vi "Format_Request.vi"(8 "error in (no error)":errorcluster, 10 "Request":T1=enum."PATCH_MULTIPART", 11 "Request in":refnum<class "Request.lvclass">) -> (0 "error out":errorcluster, 3 "Request out":refnum<class "Request.lvclass">)   [LabVIEW 2016, in "Request.lvclass"]
uses:
  Request.lvclass
  PowerShell_Format/Request_Control.ctl
  Request.lvclass/Request.ctl
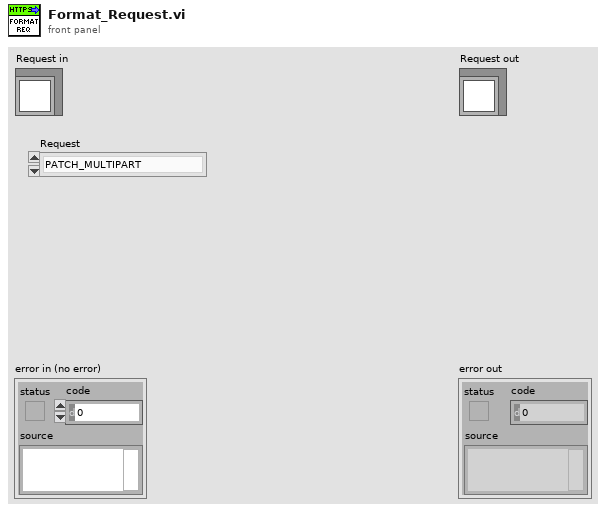
[diagram p1: front panel]
types:
  T1 = typedef "Request.lvclass/Request_Control.ctl" = enum16{"POST", "PATCH_MULTIPART", "POST_MULTIPART", "PATCH", "DELETE", "HEAD", "PUT", "GET"}
  T2 = cluster{"Name":string, "Value":string, "File":path, "Filename":string, "MIME type":string}[]
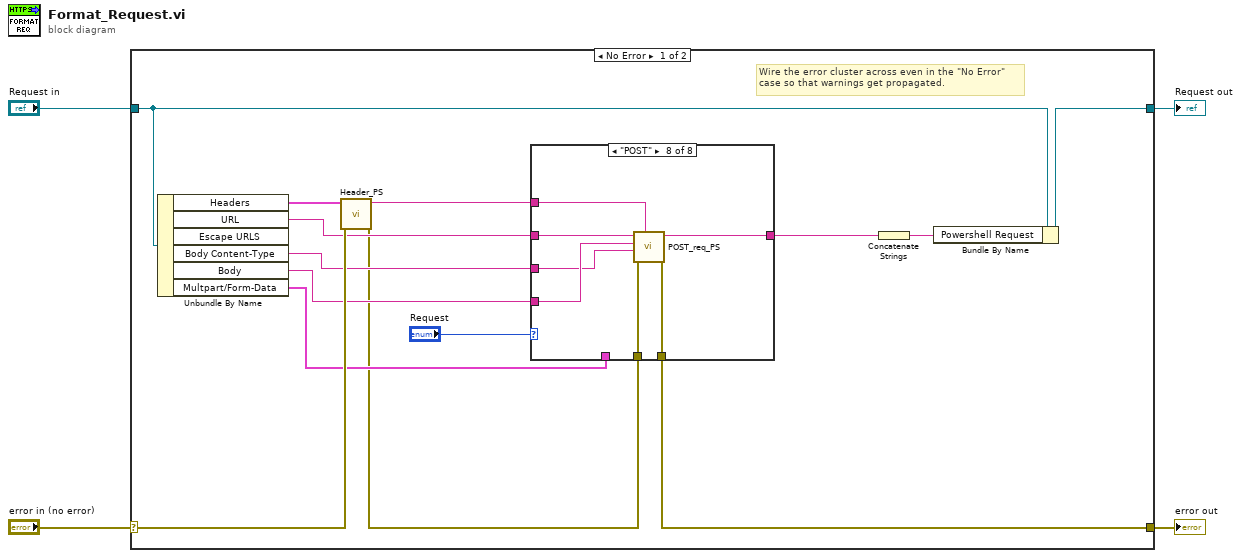
[diagram p0: block diagram]
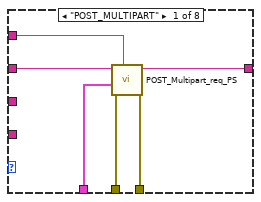
[diagram p2: hidden frame]
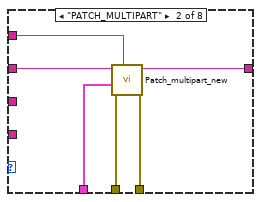
[diagram p3: hidden frame]
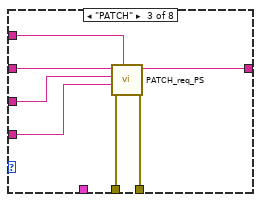
[diagram p4: hidden frame]
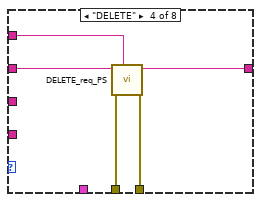
[diagram p5: hidden frame]
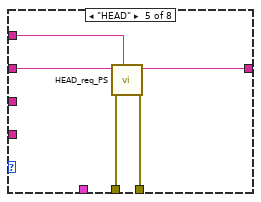
[diagram p6: hidden frame]
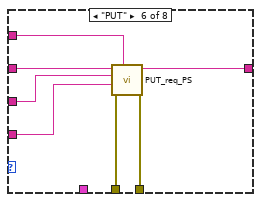
[diagram p7: hidden frame]
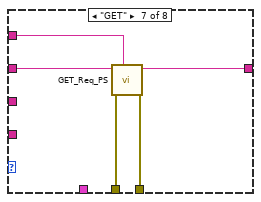
[diagram p8: hidden frame]
diagram:
  n1 = case shown="No Error" "error in (no error)" {
    selector: "error in (no error)" -> [w15 w68]
    tunnel: [w13 w68] -> w3
    tunnel: [w11 w67] -> w1
    tunnel: "Request in" -> [w12 w67]
    frame No Error {
      # "Wire the error cluster across even in the \"No Error\"\ncase so that warnings get propagated."
      n2 = Unbundle By Name(w12) -> ("Headers"=w14:cluster{"Name":string, "Value":string}[], "URL"=w9:string, "Body Content-Type"=w6:string, "Body"=w7:string, "Multpart/Form-Data"=w8:T2)  [unwired: 1 out]
      n3 = call "Header_PS.vi"("error in"=w15, "Headers In"=w14) -> ("error out"=w5:errorcluster, "Headers_PS_Dict"=w16:string)  [unwired: 8 in]
      n4 = case shown="\"POST\"" "Request" {
        tunnel: w8 -> [w24 w25 _ _ _ _ _ _]
        tunnel: w9 -> [w21 w29 w37 w39 w45 w54 w56 w62]
        tunnel: w5 -> [w23 w27 w36 w42 w47 w51 w57 w65]
        tunnel: [w22 w26 w35 w41 w46 w50 w58 w64] -> w13
        tunnel: w16 -> [w20 w30 w34 w38 w44 w49 w55 w63]
        tunnel: [w19 w28 w31 w40 w43 w48 w59 w66] -> w17
        tunnel: w6 -> [_ _ w32 _ _ w53 _ w60]
        tunnel: w7 -> [_ _ w33 _ _ w52 _ w61]
        frame "POST_MULTIPART" {
          n5 = call "POST_Multipart_req_PS.vi"("Headers"=w20, "error in"=w23, "Multpart/Form-Data"=w24, "URL"=w21) -> ("error out"=w22:errorcluster, "Multipart PATCH Request"=w19:string)  [unwired: 6 in]
        }
        frame "PATCH_MULTIPART" {
          n6 = call "Patch_multipart_new.vi"("Headers"=w30, "error in"=w27, "Multpart/Form-Data"=w25, "URL"=w29) -> ("error out"=w26:errorcluster, "Multipart PATCH Request"=w28:string)  [unwired: 6 in]
        }
        frame "PATCH" {
          n7 = call "PATCH_req_PS.vi"("Headers"=w34, "error in"=w36, "Body"=w33, "ContentType"=w32, "URL"=w37) -> ("error out"=w35:errorcluster, "PATCH Request"=w31:string)  [unwired: 5 in]
        }
        frame "DELETE" {
          n8 = call "DELETE_req_PS.vi"("Headers"=w38, "error in"=w42, "URL"=w39) -> ("error out"=w41:errorcluster, "DELETE Request"=w40:string)  [unwired: 7 in]
        }
        frame "HEAD" {
          n9 = call "HEAD_req_PS.vi"("Headers"=w44, "error in"=w47, "URL"=w45) -> ("error out"=w46:errorcluster, "HEAD Request"=w43:string)  [unwired: 7 in]
        }
        frame "PUT" {
          n10 = call "PUT_req_PS.vi"("Headers"=w49, "error in"=w51, "ContentType"=w52, "Body"=w53, "URL"=w54) -> ("error out"=w50:errorcluster, "PUT Request"=w48:string)  [unwired: 5 in]
        }
        frame "GET" {
          n11 = call "GET_Req_PS.vi"("Headers"=w55, "error in"=w57, "URL"=w56) -> ("error out"=w58:errorcluster, "GET Request"=w59:string)  [unwired: 7 in]
        }
        frame "POST" {
          n12 = call "POST_req_PS.vi"("Headers"=w63, "error in"=w65, "ContentType"=w60, "Body"=w61, "URL"=w62) -> ("error out"=w64:errorcluster, "POST Request"=w66:string)  [unwired: 5 in]
        }
      }
      n13 = Concatenate Strings(w17) -> (w10:string)
      n14 = Bundle By Name(cluster=w12, "Powershell Request"=w10) -> (w11:refnum<class "Request.lvclass">)
    }
    frame Error {
    }
  }
  "error out" <- w3
  "Request out" <- w1
